vi "TCP-Set Multipliers.vi"(8 "error in (no error)":errorcluster, 10 "Multiplier String":string, 11 "Channel String":string) -> (0 "error out":errorcluster)   [LabVIEW 2015]
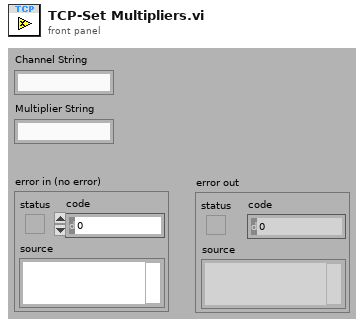
[diagram p1: front panel]
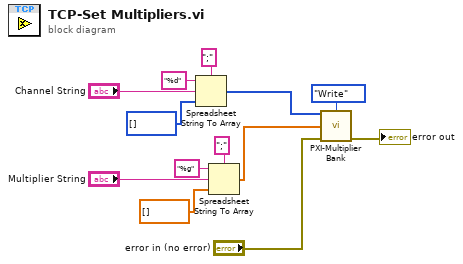
[diagram p0: block diagram]
diagram:
  n1 = Spreadsheet String To Array(delimiter (Tab)=";", format string="%d", spreadsheet string="Channel String", array type (2D Dbl)=i32[] []) -> (array=w5:i32[])
  n2 = Spreadsheet String To Array(delimiter (Tab)=";", format string="%g", spreadsheet string="Multiplier String", array type (2D Dbl)=dbl[] []) -> (array=w4:dbl[])
  n3 = call "PXI-Multiplier Bank.vi"("AO Channels"=w5, "Action"=enum16{"Init", "Write", "Read"}."Write", "Multipliers"=w4, "error in (no error)"="error in (no error)") -> ("error out"=→"error out":errorcluster)  [unwired: 9 in, 2 out]
